vi "configuration UI.vi"() -> ()   [LabVIEW 2013, in "TDMS datalogger editor node.lvclass"]
uses:
  TDMS datalogger editor node.lvclass
  <vilib>/CEF_TreeControl/Node/NodeRef.ctl
  <vilib>/CEF_TreeControl/Node/NISE_CEF_Node.lvclass
  <vilib>/NI/AMC/Message Queue.ctl
  <vilib>/NI/AMC/Message.ctl
  <vilib>/NI/Tools/Keyed Array/KeyedArray.ctl
  <vilib>/CEF_TreeControl/Node/UserEventRef.ctl
  <vilib>/CEF_TreeControl/Controls/EventCluster.ctl
  <vilib>/NI/TBM Modules/TDMS Datalogger/module/configuration/TDMS datalogger configuration.lvclass
  <vilib>/NI/Module Execution Interface/Engine Configuration/engine configuration.lvclass
  <vilib>/NI/Tag Bus Data Framework/Configuration Editor/Classes/Engine Parent/Engine Parent Editor Node.lvclass
  <vilib>/NI/Tag Bus/tag/tag descriptor.lvclass
  <vilib>/NI/Tag Bus/tag/Data Type.ctl
  <vilib>/NI/Tag Bus/tag/tag descriptor.lvclass/tag descriptor.ctl
  <vilib>/NI/Tag Bus Module Framework/root configuration/TBM configuration.lvclass/TBM configuration.ctl
  <vilib>/NI/TBM Modules/TDMS Datalogger/module/configuration/TDMS datalogger configuration.lvclass/TDMS datalogger configuration.ctl
  <vilib>/NI/Tag Bus/tag/write tag name.vi
  <vilib>/NI/Tag Bus/tag/write data type.vi
  <vilib>/NI/TBM Modules/TDMS Datalogger/module/configuration/Write scans per write.vi
  <vilib>/NI/TBM Modules/TDMS Datalogger/module/configuration/Write queue size.vi
  <vilib>/NI/TBM Modules/TDMS Datalogger/module/configuration/Write Path.vi
  <vilib>/NI/TBM Modules/TDMS Datalogger/module/configuration/Write backup directory.vi
  <vilib>/NI/TBM Modules/TDMS Datalogger/module/configuration/Write channel pattern matches.vi
  <vilib>/NI/TBM Modules/TDMS Datalogger/module/configuration/Write add enable channel.vi
  <vilib>/NI/Tag Bus Module Framework/root configuration/Read instance name.vi
  <vilib>/NI/TBM Modules/TDMS Datalogger/module/configuration/Read backup directory.vi
  <vilib>/NI/TBM Modules/TDMS Datalogger/module/configuration/Read Path.vi
  <vilib>/NI/TBM Modules/TDMS Datalogger/module/configuration/Read queue size.vi
  <vilib>/NI/TBM Modules/TDMS Datalogger/module/configuration/Read scans per write.vi
  <vilib>/NI/TBM Modules/TDMS Datalogger/module/configuration/Read add enable channel.vi
  <vilib>/NI/TBM Modules/TDMS Datalogger/module/configuration/Read channel pattern matches.vi
  <vilib>/NI/Tag Bus Data Framework/Configuration Editor/Classes/Module editor node/Read Module Configuration.vi
  <vilib>/NI/Tag Bus Module Framework/root configuration/create GUID.vi
  <vilib>/NI/Tag Bus Data Framework/Configuration Editor/Classes/Module editor node/Write Module Configuration.vi
  <vilib>/NI/Tag Bus Data Framework/Configuration Editor/Classes/Engine Parent/write engine configuration.vi
  <vilib>/NI/Tag Bus Module Framework/root configuration/TBM configuration.lvclass
  <vilib>/NI/Tag Bus Module Framework/module configuration/TBM module configuration.lvclass
  <vilib>/NI/Tag Bus Data Framework/Configuration Editor/Classes/Module editor node/module editor node.lvclass
  <vilib>/CEF_TreeControl/NISE_CEF_TreeControl.lvlib
  <vilib>/NI/Tools/Keyed Array/Tools_KeyedArray.lvlib
  <vilib>/NI/AMC/AMC.lvlib
panel:
  in  "Tab Control":T1(tab)
  in  "channels":i32(listbox)
  in  "remove":bool
  in  "avail tags":i32(listbox)=-1
  in  "add all":bool
  in  "add1":bool
  out "Enable Tag":string
  in  "history error":bool
  in  "path error":bool
  in  "Historical Directory":path
  in  "use enable channel":bool
  in  "recalc":bool
  out "Approximate memory usage":dbl
  in  "queue size":i32=2
  in  "scans per write":i32=20
  in  "File Path":path
  in  "Channel Subscription Pattern Matches":string[](array[string])
  in  "Enable Dynamic Mapping":bool
  in  "user event":T2
  in  "main queue":T3
  in  "node ref":T4
  # "kB"
  # "Note: This value ignores dynamic mapping"
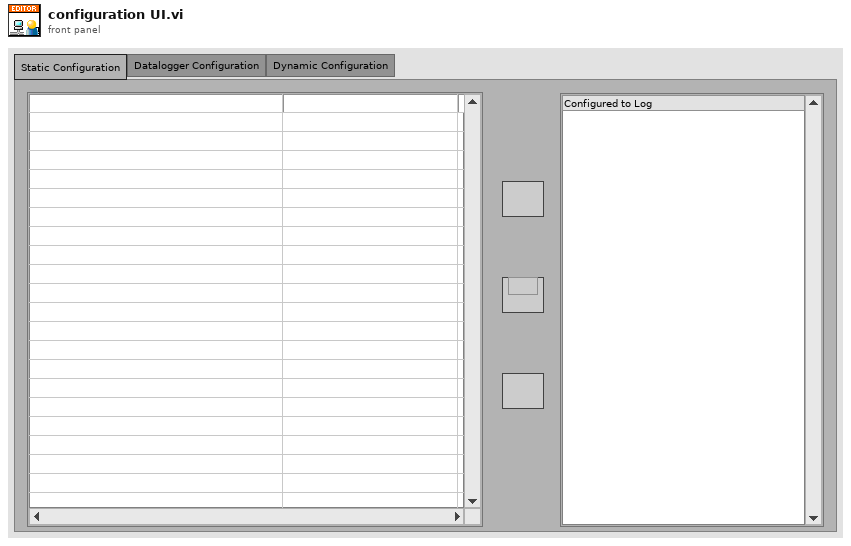
[diagram p1: front panel]
types:
  T1 = enum32{"Static Configuration", "Datalogger Configuration", "Dynamic Configuration"}
  T2 = typedef "NISE_CEF_Node.lvclass/UserEventRef.ctl" = refnum<user-event>
  T3 = typedef "AMC.lvlib/Message Queue.ctl" = refnum<queue>
  T4 = typedef "NISE_CEF_Node.lvclass/NodeRef.ctl" = refnum<data-value>
  T5 = typedef "tag bus.lvlib/tag descriptor.lvclass/Data Type.ctl" = enum16{"Double", "Single", "I64", "I32", "I16", "I8", "U64", "U32", "U16", "U8", "Boolean", "String", "Array of Double", "Array of Single", "Array of I64", "Array of I32", "Array of I16", "Array of I8", "Array of U64", "Array of U32", "Array of U16", "Array of U8", "Array of Boolean", "Array of String"}
  T6 = typedef "NISE_CEF_TreeControl.lvlib/EventCluster.ctl" = cluster{"command":string, "data":string}
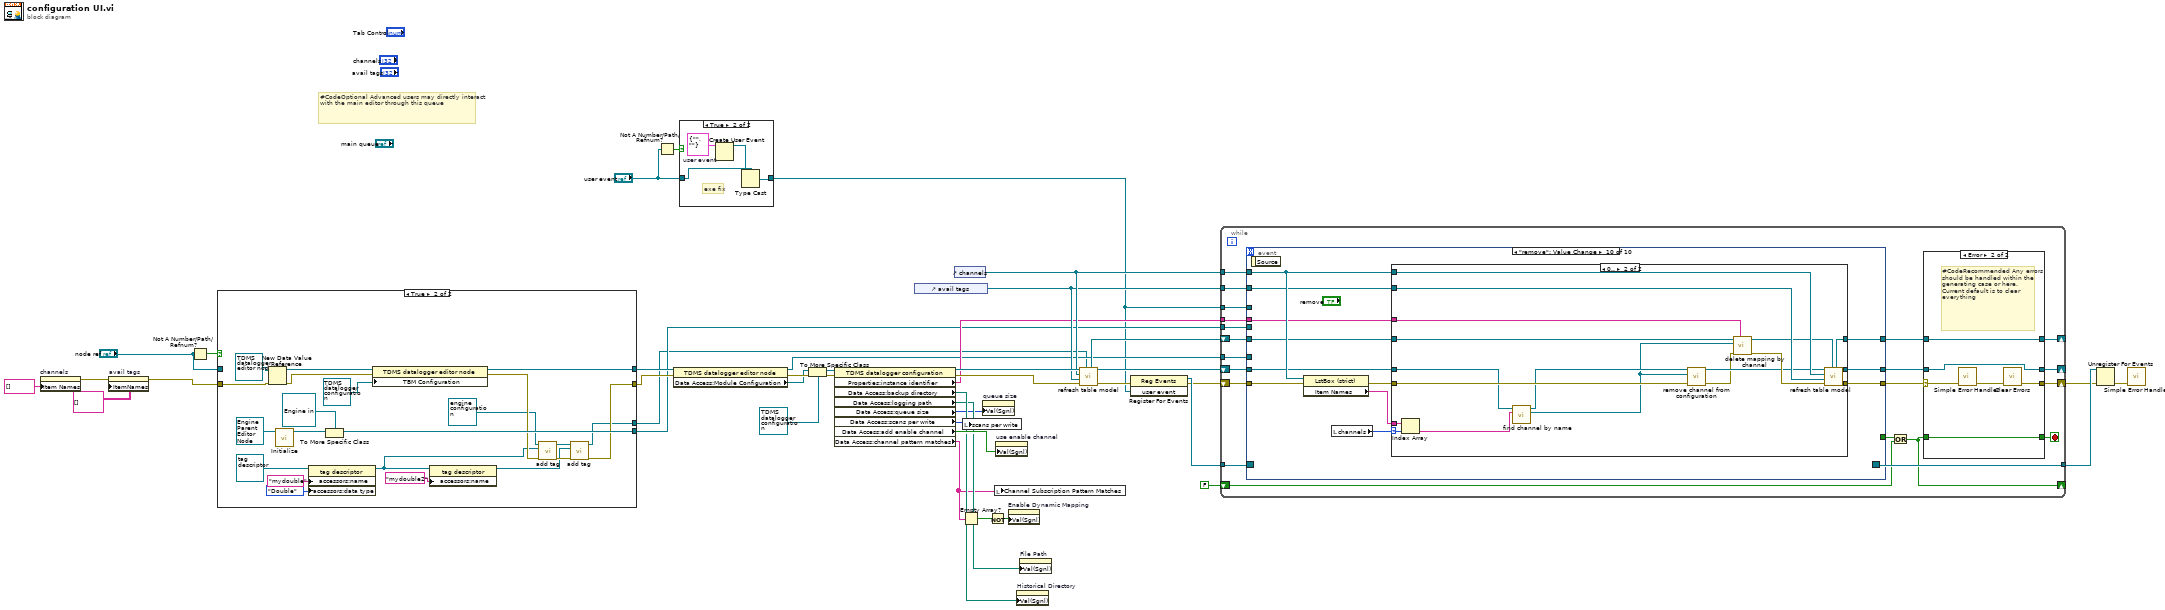
[diagram p0: block diagram]
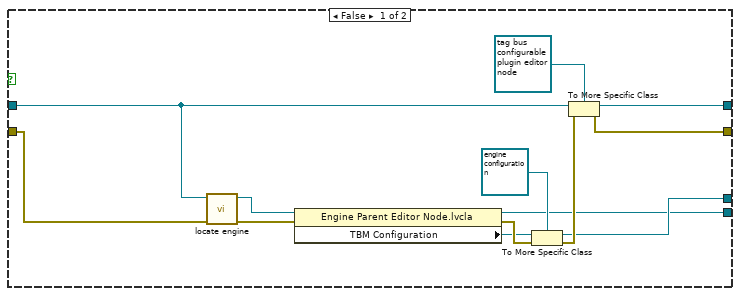
[diagram p2: hidden frame]
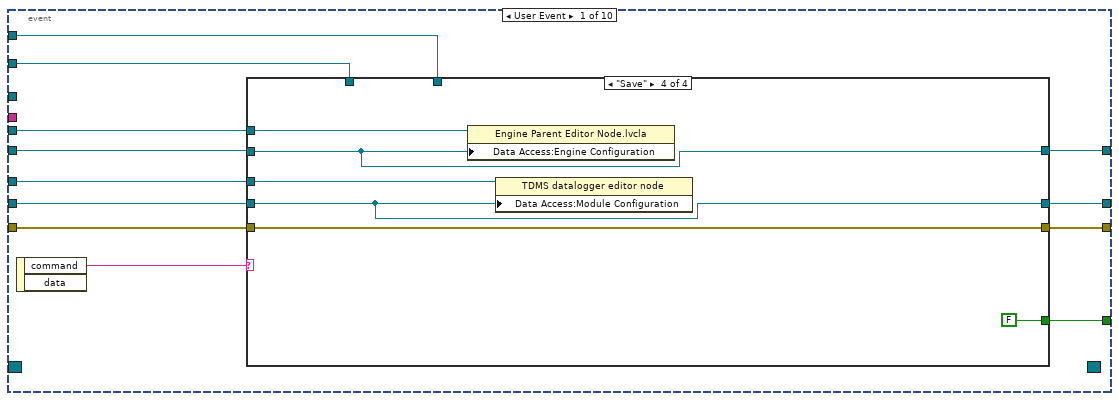
[diagram p5: hidden frame]
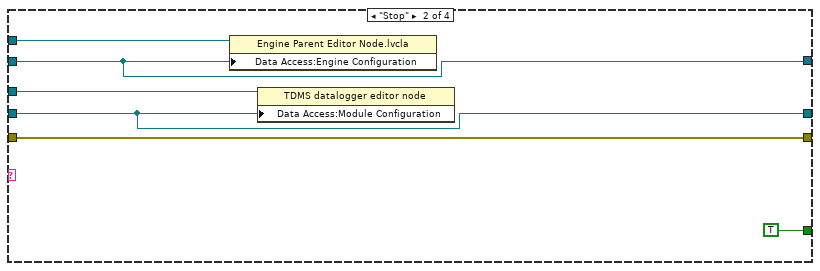
[diagram p7: hidden frame]
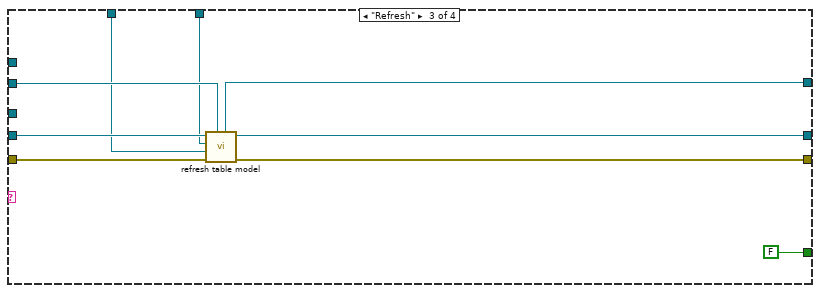
[diagram p8: hidden frame]
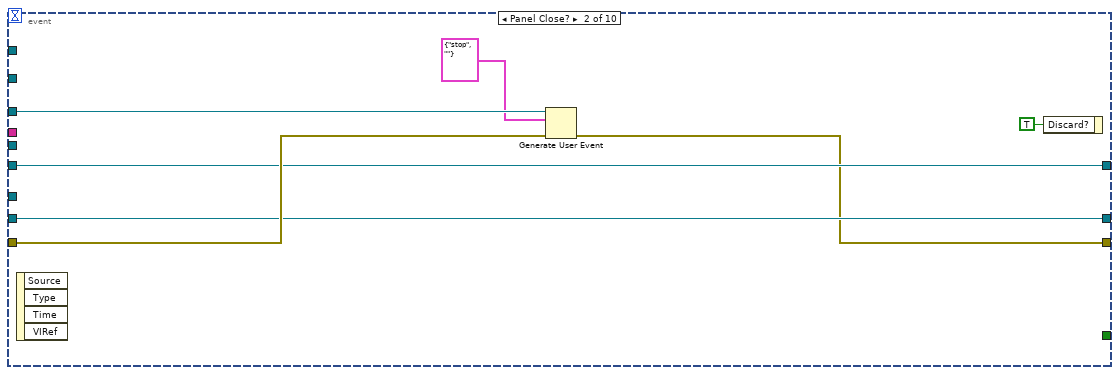
[diagram p9: hidden frame]
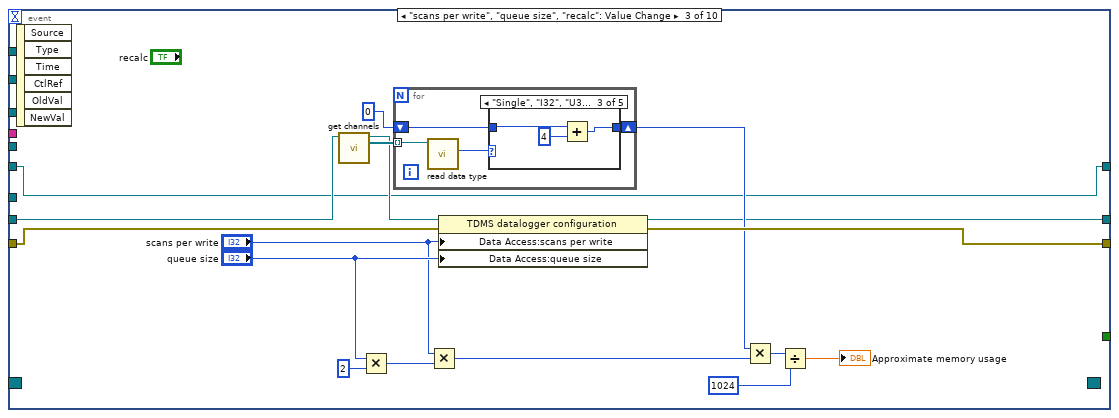
[diagram p10: hidden frame]
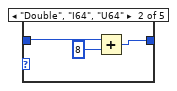
[diagram p12: hidden frame]
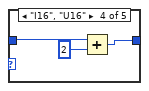
[diagram p13: hidden frame]
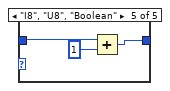
[diagram p14: hidden frame]
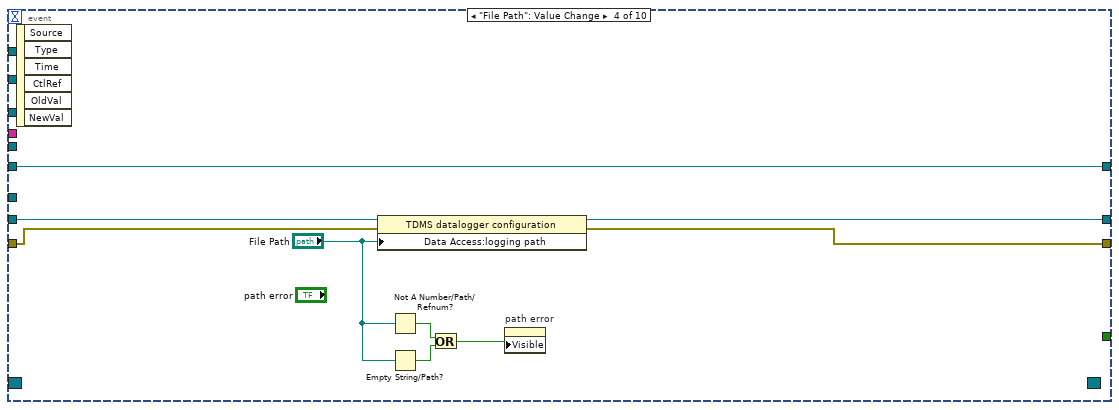
[diagram p15: hidden frame]
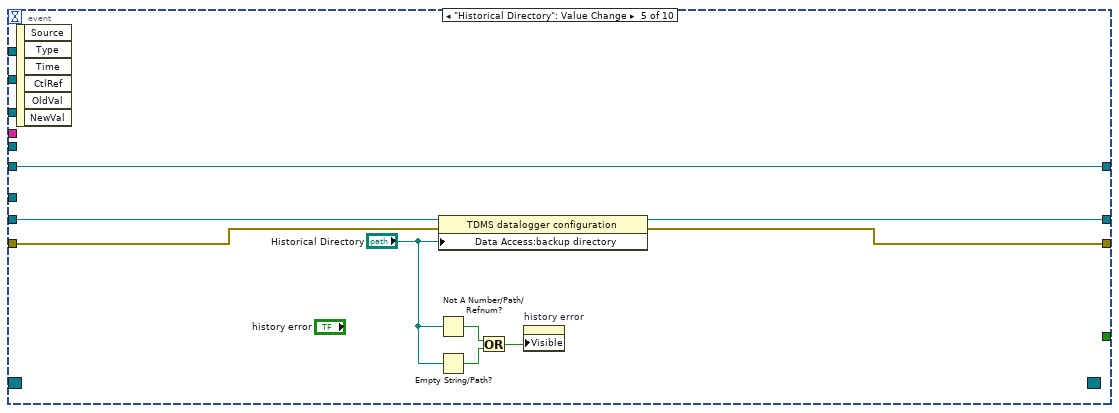
[diagram p16: hidden frame]
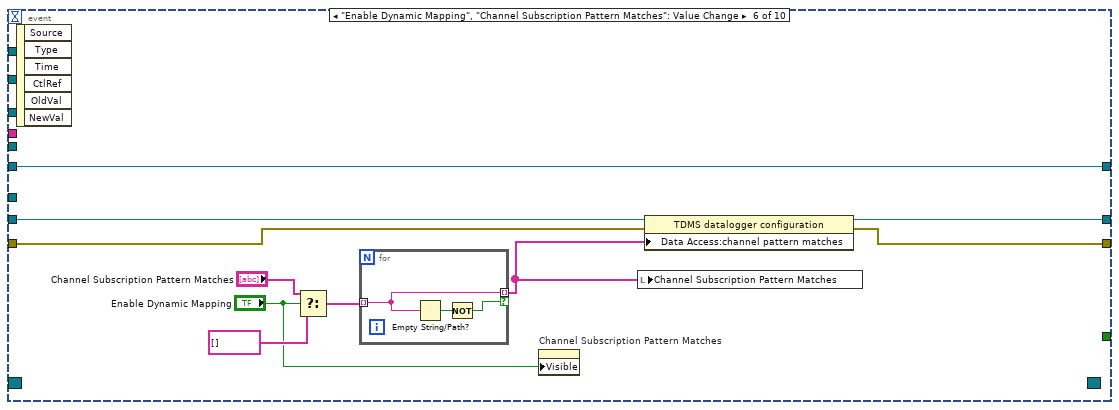
[diagram p17: hidden frame]
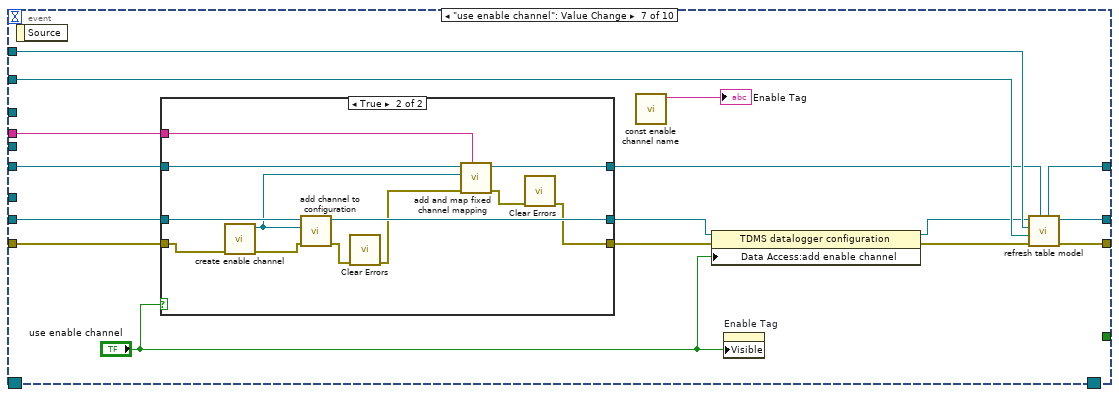
[diagram p18: hidden frame]
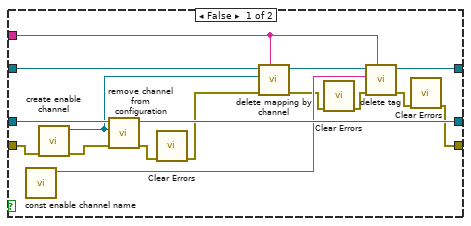
[diagram p19: hidden frame]
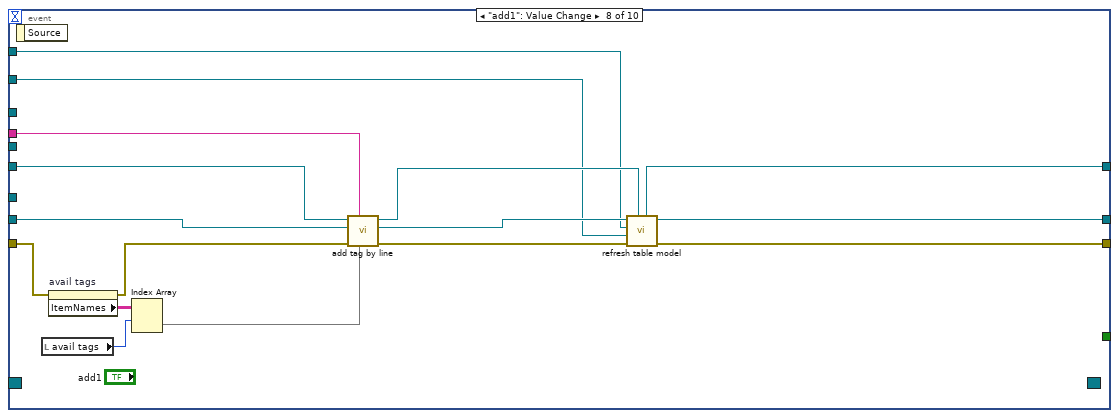
[diagram p20: hidden frame]
diagram:
  # "#CodeOptional Advanced users may directly interact with the main editor through this queue"
  n1 = property on="channels" class="LstBox (strict)"("Item Names"=string[] []) -> (error out=w15:errorcluster)  [unwired: 2 in, 1 out]
  n2 = property on="avail tags" class="MCListbox (strict)"(error in=w15, "ItemNames"=string[][] [] ("Item Names")) -> (error out=w4:errorcluster)  [unwired: 1 in, 1 out]
  n3 = Not A Number/Path/Refnum?(number/path/refnum="node ref") -> (NaN/Path/Refnum?=w6:bool)
  n4 = case shown="True" w6 {
    tunnel: "node ref" -> [w53 _]
    tunnel: [w52 w76] -> w8
    tunnel: [w51 w63] -> w7
    tunnel: [w44 w62] -> w2
    tunnel: [w43 w73] -> w3
    tunnel: w4 -> [w42 w55]
    frame False {
      n5 = call <vilib>:"locate engine.vi"("error in"=w42, "component"=w53) -> ("error out"=w48:errorcluster, "engine"=w50:refnum<data-value>)  [unwired: 8 in]
      n6 = property class="Engine Parent Editor Node.lvcla"(reference=w50, error in=w48) -> (reference out=w43:refnum<data-value>, error out=w47:errorcluster, "TBM Configuration"=w46:refnum<class "TBM configuration.lvclass">)
      n7 = To More Specific Class(target class=refnum<class "engine configuration.lvclass"> refnum ("engine configuration.lvclass"), reference=w46, error in=w47) -> (specific class reference=w44:refnum<class "engine configuration.lvclass">, error out=w45:errorcluster)
      n8 = To More Specific Class(target class=refnum<data-value> refnum ("data value reference"), reference=w53, error in=w45) -> (specific class reference=w52:refnum<data-value>, error out=w51:errorcluster)
    }
    frame True {
      n9 = New Data Value Reference(data value=refnum<class "TDMS datalogger editor node.lvclass"> refnum ("tag bus configurable plugin editor node"), error in=w55) -> (data value reference=w75:refnum<data-value>, error out=w56:errorcluster)
      n10 = call-dynamic "Initialize.vi"("Engine in"=refnum<class "Engine Parent Editor Node.lvclass"> refnum) -> ("data value reference"=w74:T4)  [unwired: 8 in, 2 out]
      n11 = property class="tag descriptor"(reference=refnum<class "tag descriptor.lvclass"> refnum ("tag descriptor"), "accessors:name"="mydouble" ("name"), "accessors:data type"=Data_Type."Double" ("data type")) -> (reference out=w60:refnum<class "tag descriptor.lvclass">)  [unwired: 1 in, 1 out]
      n12 = To More Specific Class(target class=refnum<data-value> refnum ("data value reference"), reference=w74) -> (specific class reference=w73:refnum<data-value>)  [unwired: 1 in, 1 out]
      n13 = property class="TDMS datalogger editor node"(reference=w75, error in=w56, "TBM Configuration"=refnum<class "TDMS datalogger configuration.lvclass"> refnum ("TDMS datalogger configuration")) -> (reference out=w76:refnum<data-value>, error out=w67:errorcluster)
      n14 = property class="tag descriptor"(reference=w60, "accessors:name"="mydouble2" ("name")) -> (reference out=w61:refnum<class "tag descriptor.lvclass">)  [unwired: 1 in, 1 out]
      n15 = call <vilib>:"add tag.vi"("error in"=w67, "tag descriptor"=w60, "engine configuration in"=refnum<class "engine configuration.lvclass"> refnum ("Engine Configuration")) -> ("error out"=w65:errorcluster, "engine configuration out"=w64:refnum<class "engine configuration.lvclass">)  [unwired: 7 in]
      n16 = call <vilib>:"add tag.vi"("error in"=w65, "tag descriptor"=w61, "engine configuration in"=w64) -> ("error out"=w63:errorcluster, "engine configuration out"=w62:refnum<class "engine configuration.lvclass">)  [unwired: 7 in]
    }
  }
  n17 = Not A Number/Path/Refnum?(number/path/refnum="user event") -> (NaN/Path/Refnum?=w10:bool)
  n18 = property class="TDMS datalogger editor node"(reference=w8, error in=w7) -> (reference out=w11:refnum<data-value>, error out=w36:errorcluster, "Data Access:Module Configuration"=w26:refnum<class "TBM module configuration.lvclass">)
  n19 = case shown="True" w10 {
    tunnel: [w77 w80] -> w1
    tunnel: "user event" -> [w77 w81]
    frame False {
    }
    frame True {
      w78 = T6 {"command"="", "data"=""}  # user event
      # "exe fix"
      n20 = Create User Event(user event datatype=w78) -> (user event=w79:refnum<user-event>)  [unwired: 1 in, 1 out]
      n21 = Type Cast(type=w81, x=w79) -> (*(type *) &x=w80:T2)
    }
  }
  n22 = To More Specific Class(target class=refnum<class "TDMS datalogger configuration.lvclass"> refnum ("TDMS datalogger configuration"), reference=w26, error in=w36) -> (specific class reference=w24:refnum<class "TDMS datalogger configuration.lvclass">, error out=w27:errorcluster)
  n23 = property class="TDMS datalogger configuration"(reference=w24, error in=w27) -> (reference out=w20:refnum<class "TDMS datalogger configuration.lvclass">, error out=w19:errorcluster, "Properties:instance identifier"=w16:string, "Data Access:backup directory"=w33:path, "Data Access:logging path"=w32:path, "Data Access:queue size"=w31:i32, "Data Access:scans per write"=w35:i32, "Data Access:add enable channel"=w34:bool, "Data Access:channel pattern matches"=w30:string[])
  n24 = control-ref of="avail tags"() -> (w17:refnum<vi>)
  n25 = control-ref of="channels"() -> (w18:refnum<vi>)
  n26 = Empty Array?(array=w30) -> (empty?=w28:bool)
  n27 = local write "scans per write"(w35) -> ()
  n28 = property on="queue size" class="DigNum (strict)"("Val(Sgnl)"=w31) -> ()  [unwired: 2 in, 2 out]
  n29 = Not(x=w28) -> (.not. x?=w29:bool)
  n30 = local write "Channel Subscription Pattern Matches"(w30) -> ()
  n31 = property on="use enable channel" class="Bool (strict)"("Val(Sgnl)"=w34) -> ()  [unwired: 2 in, 2 out]
  n32 = property on="Enable Dynamic Mapping" class="Bool (strict)"("Val(Sgnl)"=w29) -> ()  [unwired: 2 in, 2 out]
  n33 = property on="Historical Directory" class="Path"("Val(Sgnl)"=w33) -> ()  [unwired: 2 in, 2 out]
  n34 = property on="File Path" class="Path"("Val(Sgnl)"=w32) -> ()  [unwired: 2 in, 2 out]
  n35 = call "refresh table model.vi"("engine configuration"=w2, "error in"=w19, "avail tags"=w17, "chan table"=w18, "TDMS datalogger configuration"=w20) -> ("error out"=w23:errorcluster, "TDMS datalogger configuration out"=w22:refnum<class "TDMS datalogger configuration.lvclass">, "engine configuration out"=w21:refnum<class "engine configuration.lvclass">)  [unwired: 4 in]
  n36 = register-events(error in=w23, w1) -> (reference out=w41:refnum<event-registration>, error out=w38:errorcluster)  [unwired: 1 in]
  n37 = while {
    tunnel: w41 -> [w102]
    tunnel: [w101] -> w40
    shift-right: [w94] -> w12
    shift-left: w38 -> [w100]
    shift-right: [w96] -> _
    shift-left: FALSE -> [w95]
    shift-right: [w91] -> _
    shift-left: w22 -> [w93]
    shift-right: [w89] -> _
    shift-left: w21 -> [w90]
    tunnel: w18 -> [w87]
    tunnel: w17 -> [w86]
    tunnel: w16 -> [w85]
    tunnel: w3 -> [w84]
    tunnel: w11 -> [w83]
    tunnel: w1 -> [w82]
    stop <- w98 stop-if-true
    n38 = event shown="[9] \"remove\": Value Change" {
      selector: w102 -> [_ _ _ _ _ _ _ _ _ _]
      dyn-events: [_ _ _ _ _ _ _ _ _ _] -> w101
      timeout: _ -> [_ _ _ _ _ _ _ _ _ _]
      tunnel: [w124 _ _ _ _ _ _ _ _ _] -> w97
      tunnel: [w122 w151 w171 w196 w205 w215 w236 w275 w290 w314] -> w99
      tunnel: w100 -> [w121 w155 w172 w198 w207 w217 w224 w280 w292 w313]
      tunnel: w93 -> [w119 w154 w159 w197 w206 w216 w225 w265 w291 w304]
      tunnel: [w115 w154 w157 w191 w200 w211 w235 w274 w286 w307] -> w92
      tunnel: [w116 w153 w156 w190 w199 w210 w234 w273 w287 w306] -> w88
      tunnel: w90 -> [w120 w153 w156 w190 w199 w210 w227 w267 w283 w308]
      tunnel: w87 -> [w114 _ _ _ _ _ w233 w270 w284 w311]
      tunnel: w86 -> [w113 _ _ _ _ _ w232 w269 w285 w310]
      tunnel: w85 -> [_ _ _ _ _ _ w229 w268 w281 w305]
      tunnel: w84 -> [w118 _ _ _ _ _ _ _ _ _]
      tunnel: w83 -> [w117 _ _ _ _ _ _ _ _ _]
      tunnel: w82 -> [_ w150 _ _ _ _ _ _ _ _]
      event User Event {
        n39 = event-data() -> ("command"=w123:string)  [unwired: 1 in, 1 out]
        n40 = case shown="\"Save\"" w123 {
          tunnel: [_ TRUE FALSE FALSE] -> w124
          tunnel: [w127 w132 w140 w147] -> w122
          tunnel: w121 -> [w127 w132 w141 w147]
          tunnel: w120 -> [w126 w131 w139 w146]
          tunnel: w119 -> [w125 w130 w137 w145]
          tunnel: w118 -> [_ w128 _ w143]
          tunnel: w117 -> [_ w129 _ w144]
          tunnel: [w126 w131 w138 w146] -> w116
          tunnel: [w125 w130 w136 w145] -> w115
          tunnel: w114 -> [_ _ w135 _]
          tunnel: w113 -> [_ _ w134 _]
          frame Default {
          }
          frame "Stop" {
            n41 = property class="Engine Parent Editor Node.lvcla"(reference=w128, "Data Access:Engine Configuration"=w131) -> ()  [unwired: 1 in, 2 out]
            n42 = property class="TDMS datalogger editor node"(reference=w129, "Data Access:Module Configuration"=w130) -> ()  [unwired: 1 in, 2 out]
          }
          frame "Refresh" {
            n43 = call "refresh table model.vi"("engine configuration"=w139, "error in"=w141, "avail tags"=w134, "chan table"=w135, "TDMS datalogger configuration"=w137) -> ("error out"=w140:errorcluster, "TDMS datalogger configuration out"=w136:refnum<class "TDMS datalogger configuration.lvclass">, "engine configuration out"=w138:refnum<class "engine configuration.lvclass">)  [unwired: 4 in]
          }
          frame "Save" {
            n44 = property class="Engine Parent Editor Node.lvcla"(reference=w143, "Data Access:Engine Configuration"=w146) -> ()  [unwired: 1 in, 2 out]
            n45 = property class="TDMS datalogger editor node"(reference=w144, "Data Access:Module Configuration"=w145) -> ()  [unwired: 1 in, 2 out]
          }
        }
      }
      event Panel Close? {
        n46 = event-data() -> ()  [unwired: 1 in, 4 out]
        n47 = Generate User Event(user event=w150, event data cluster=T6 {"command"="stop", "data"=""} ("event data"), error in=w155) -> (error out=w151:errorcluster)  [unwired: 1 in, 1 out]
        n48 = event-data("Discard?"=TRUE) -> ()  [unwired: 1 in, 1 out]
      }
      event "scans per write", "queue size", "recalc": Value Change {
        n49 = event-data() -> ()  [unwired: 1 in, 6 out]
        n50 = call-dynamic "get channels.vi"("module configuration in"=w159) -> ("channels"=w161:refnum<class "TBM channel.lvclass">[], "module configuration out"=w158:refnum<class "TDMS datalogger configuration.lvclass">)  [unwired: 9 in]
        n51 = Multiply(x="queue size", y=2 ("x")) -> (x*y=w170:i32)
        n52 = for {
          shift-right: [w175] -> w162
          shift-left: u32 0 -> [w176]
          tunnel: w161 -> [w173] mode=indexing
          n53 = call <vilib>:"read data type.vi"("system tag in"=w173) -> ("data type"=w174:T5)  [unwired: 8 in, 2 out]
          n54 = case shown="\"Single\", \"I32\", \"U32\"" w174 {
            tunnel: w176 -> [w177 w180 w183 w186 w189]
            tunnel: [w177 w179 w182 w185 w188] -> w175
            frame Default {
            }
            frame "Double", "I64", "U64" {
              n55 = Add(x=w180, y=u32 8) -> (x+y=w179:u32)
            }
            frame "Single", "I32", "U32" {
              n56 = Add(x=w183, y=u32 4) -> (x+y=w182:u32)
            }
            frame "I16", "U16" {
              n57 = Add(x=w186, y=u32 2) -> (x+y=w185:u32)
            }
            frame "I8", "U8", "Boolean" {
              n58 = Add(x=w189, y=u32 1) -> (x+y=w188:u32)
            }
          }
        }
        n59 = Multiply(x="scans per write", y=w170) -> (x*y=w164:i32)
        n60 = property class="TDMS datalogger configuration"(reference=w158, error in=w172, "Data Access:scans per write"="scans per write", "Data Access:queue size"="queue size") -> (reference out=w157:refnum<class "TDMS datalogger configuration.lvclass">, error out=w171:errorcluster)
        n61 = Multiply(x=w162, y=w164) -> (x*y=w166:u32)
        n62 = Divide(x=w166, y=u32 1024) -> (x/y=→"Approximate memory usage":dbl)
      }
      event "File Path": Value Change {
        n63 = event-data() -> ()  [unwired: 1 in, 6 out]
        n64 = property class="TDMS datalogger configuration"(reference=w197, error in=w198, "Data Access:logging path"="File Path") -> (reference out=w191:refnum<class "TDMS datalogger configuration.lvclass">, error out=w196:errorcluster)
        n65 = Not A Number/Path/Refnum?(number/path/refnum="File Path") -> (NaN/Path/Refnum?=w193:bool)
        n66 = Empty String/Path?(string/path="File Path") -> (empty?=w194:bool)
        n67 = Or(x=w193, y=w194) -> (x .or. y?=w192:bool)
        n68 = property on="path error" class="Bool"("Visible"=w192) -> ()  [unwired: 2 in, 2 out]
      }
      event "Historical Directory": Value Change {
        n69 = event-data() -> ()  [unwired: 1 in, 6 out]
        n70 = Not A Number/Path/Refnum?(number/path/refnum="Historical Directory") -> (NaN/Path/Refnum?=w203:bool)
        n71 = Empty String/Path?(string/path="Historical Directory") -> (empty?=w204:bool)
        n72 = property class="TDMS datalogger configuration"(reference=w206, error in=w207, "Data Access:backup directory"="Historical Directory") -> (reference out=w200:refnum<class "TDMS datalogger configuration.lvclass">, error out=w205:errorcluster)
        n73 = Or(x=w203, y=w204) -> (x .or. y?=w201:bool)
        n74 = property on="history error" class="Bool"("Visible"=w201) -> ()  [unwired: 2 in, 2 out]
      }
      event "Enable Dynamic Mapping", "Channel Subscription Pattern Matches": Value Change {
        n75 = event-data() -> ()  [unwired: 1 in, 6 out]
        n76 = Select(t="Channel Subscription Pattern Matches", s="Enable Dynamic Mapping", f=string[] []) -> (s? t:f=w209:string[])
        n77 = for {
          tunnel: w209 -> [w220] mode=indexing
          tunnel: [w220] -> w208 mode=indexing if=w218
          n78 = Empty String/Path?(string/path=w220) -> (empty?=w219:bool)
          n79 = Not(x=w219) -> (.not. x?=w218:bool)
        }
        n80 = property on="Channel Subscription Pattern Matches" class="Arr (strict)"("Visible"="Enable Dynamic Mapping") -> ()  [unwired: 2 in, 2 out]
        n81 = local write "Channel Subscription Pattern Matches"(w208) -> ()
        n82 = property class="TDMS datalogger configuration"(reference=w216, error in=w217, "Data Access:channel pattern matches"=w208) -> (reference out=w211:refnum<class "TDMS datalogger configuration.lvclass">, error out=w215:errorcluster)
      }
      event "use enable channel": Value Change {
        n83 = event-data() -> ()  [unwired: 1 in, 1 out]
        n84 = case shown="True" "use enable channel" {
          tunnel: w229 -> [w244 w262]
          tunnel: [w245 w263] -> w228
          tunnel: w227 -> [w248 w257]
          tunnel: [w250 w261] -> w226
          tunnel: w225 -> [w251 w260]
          tunnel: w224 -> [w252 w264]
          tunnel: [w239 w255] -> w223
          frame False {
            n85 = call <vilib>:"const enable channel name.vi"() -> ("enable channel"=w243:string)  [unwired: 11 in]
            n86 = call <vilib>:"create enable channel.vi"("error in"=w252) -> ("error out"=w249:errorcluster, "enable channel"=w247:refnum<class "TBM channel.lvclass">)  [unwired: 9 in]
            n87 = call <vilib>:"remove channel from configuration.vi"("error in"=w249, "TBM channel in"=w247, "TDMS datalogger configuration in"=w251) -> ("error out"=w238:errorcluster, "TDMS datalogger configuration out"=w250:refnum<class "TDMS datalogger configuration.lvclass">)  [unwired: 7 in]
            n88 = call <vilib>:"Clear Errors.vi"("error in (no error)"=w238) -> ("error out"=w237:errorcluster)  [unwired: 6 in]
            n89 = call <vilib>:"delete mapping by channel.vi"("owner ID"=w244, "error in"=w237, "channel"=w247, "engine configuration in"=w248) -> ("error out"=w241:errorcluster, "engine configuration out"=w246:refnum<class "engine configuration.lvclass">)  [unwired: 6 in]
            n90 = call <vilib>:"Clear Errors.vi"("error in (no error)"=w241) -> ("error out"=w242:errorcluster)  [unwired: 6 in]
            n91 = call <vilib>:"delete tag.vi"("owner ID"=w244, "error in"=w242, "tag name"=w243, "engine configuration in"=w246) -> ("error out"=w240:errorcluster, "engine configuration out"=w245:refnum<class "engine configuration.lvclass">)  [unwired: 6 in]
            n92 = call <vilib>:"Clear Errors.vi"("error in (no error)"=w240) -> ("error out"=w239:errorcluster)  [unwired: 6 in]
          }
          frame True {
            n93 = call <vilib>:"create enable channel.vi"("error in"=w264) -> ("error out"=w259:errorcluster, "enable channel"=w258:refnum<class "TBM channel.lvclass">)  [unwired: 9 in]
            n94 = call <vilib>:"add channel to configuration.vi"("error in"=w259, "TBM channel in"=w258, "TDMS datalogger configuration in"=w260) -> ("error out"=w254:errorcluster, "TDMS datalogger configuration out"=w261:refnum<class "TDMS datalogger configuration.lvclass">)  [unwired: 7 in]
            n95 = call <vilib>:"Clear Errors.vi"("error in (no error)"=w254) -> ("error out"=w253:errorcluster)  [unwired: 6 in]
            n96 = call <vilib>:"add and map fixed channel mapping.vi"("module instance"=w262, "error in"=w253, "fixed channel"=w258, "engine configuration in"=w257) -> ("error out"=w256:errorcluster, "engine configuration out"=w263:refnum<class "engine configuration.lvclass">)  [unwired: 6 in]
            n97 = call <vilib>:"Clear Errors.vi"("error in (no error)"=w256) -> ("error out"=w255:errorcluster)  [unwired: 6 in]
          }
        }
        n98 = call <vilib>:"const enable channel name.vi"() -> ("enable channel"=→"Enable Tag":string)  [unwired: 11 in]
        n99 = property class="TDMS datalogger configuration"(reference=w226, error in=w223, "Data Access:add enable channel"="use enable channel") -> (reference out=w230:refnum<class "TDMS datalogger configuration.lvclass">, error out=w231:errorcluster)
        n100 = property on="Enable Tag" class="Str"("Visible"="use enable channel") -> ()  [unwired: 2 in, 2 out]
        n101 = call "refresh table model.vi"("engine configuration"=w228, "error in"=w231, "avail tags"=w232, "chan table"=w233, "TDMS datalogger configuration"=w230) -> ("error out"=w236:errorcluster, "TDMS datalogger configuration out"=w235:refnum<class "TDMS datalogger configuration.lvclass">, "engine configuration out"=w234:refnum<class "engine configuration.lvclass">)  [unwired: 4 in]
      }
      event "add1": Value Change {
        n102 = event-data() -> ()  [unwired: 1 in, 1 out]
        n103 = local read "avail tags"() -> (w278:i32)
        n104 = property on="avail tags" class="MCListbox (strict)"(error in=w280) -> (error out=w277:errorcluster, "ItemNames"=w279:string[][])  [unwired: 1 in, 1 out]
        n105 = Index Array(array=w279, index (row)=w278) -> (element=w266:string[])  [unwired: 1 in]
        n106 = call "add tag by line.vi"("ItemNames"=w266, "Properties:instance identifier"=w268, "error in"=w277, "TDMS datalogger configuration in"=w265, "engine configuration in"=w267) -> ("error out"=w276:errorcluster, "TDMS datalogger configuration out"=w271:refnum<class "TDMS datalogger configuration.lvclass">, "engine configuration out"=w272:refnum<class "engine configuration.lvclass">)  [unwired: 4 in]
        n107 = call "refresh table model.vi"("engine configuration"=w272, "error in"=w276, "avail tags"=w269, "chan table"=w270, "TDMS datalogger configuration"=w271) -> ("error out"=w275:errorcluster, "TDMS datalogger configuration out"=w274:refnum<class "TDMS datalogger configuration.lvclass">, "engine configuration out"=w273:refnum<class "engine configuration.lvclass">)  [unwired: 4 in]
      }
      event "add all": Value Change {
        n108 = event-data() -> ()  [unwired: 1 in, 1 out]
        n109 = property on="avail tags" class="MCListbox (strict)"(error in=w292) -> (error out=w294:errorcluster, "ItemNames"=w293:string[][])  [unwired: 1 in, 1 out]
        n110 = for {
          tunnel: w293 -> [w295] mode=indexing
          shift-right: [w301] -> w289
          shift-left: w294 -> [w299]
          shift-right: [w302] -> w288
          shift-left: w291 -> [w300]
          shift-right: [w297] -> w282
          shift-left: w283 -> [w298]
          tunnel: w281 -> [w296]
          n111 = call "add tag by line.vi"("ItemNames"=w295, "Properties:instance identifier"=w296, "error in"=w299, "TDMS datalogger configuration in"=w300, "engine configuration in"=w298) -> ("error out"=w301:errorcluster, "TDMS datalogger configuration out"=w302:refnum<class "TDMS datalogger configuration.lvclass">, "engine configuration out"=w297:refnum<class "engine configuration.lvclass">)  [unwired: 4 in]
        }
        n112 = call "refresh table model.vi"("engine configuration"=w282, "error in"=w289, "avail tags"=w285, "chan table"=w284, "TDMS datalogger configuration"=w288) -> ("error out"=w290:errorcluster, "TDMS datalogger configuration out"=w286:refnum<class "TDMS datalogger configuration.lvclass">, "engine configuration out"=w287:refnum<class "engine configuration.lvclass">)  [unwired: 4 in]
      }
      event "remove": Value Change {
        n113 = event-data() -> ()  [unwired: 1 in, 1 out]
        n114 = property class="LstBox (strict)"(reference=w311, error in=w313) -> (error out=w309:errorcluster, "Item Names"=w312:string[])  [unwired: 1 out]
        n115 = local read "channels"() -> (w303:i32)
        n116 = case shown="0.." w303 {
          selector: w303 -> [_ w318]
          tunnel: [w315 w335] -> w314
          tunnel: w312 -> [_ w334]
          tunnel: w311 -> [_ w333]
          tunnel: w310 -> [_ w332]
          tunnel: w309 -> [w315 w331]
          tunnel: w308 -> [w317 w330]
          tunnel: [w316 w327] -> w307
          tunnel: [w317 w325] -> w306
          tunnel: w305 -> [_ w324]
          tunnel: w304 -> [w316 w322]
          frame ..-1 {
          }
          frame 0.. {
            n117 = Index Array(array=w334, index=w318) -> (element=w320:string)
            n118 = call <vilib>:"find channel by name.vi"("channel name"=w320, "TDMS datalogger configuration in"=w322) -> ("channel"=w319:refnum<class "TBM channel.lvclass">, "TDMS datalogger configuration out"=w321:refnum<class "TDMS datalogger configuration.lvclass">)  [unwired: 8 in]
            n119 = call <vilib>:"remove channel from configuration.vi"("error in"=w331, "TBM channel in"=w319, "TDMS datalogger configuration in"=w321) -> ("error out"=w323:errorcluster, "TDMS datalogger configuration out"=w328:refnum<class "TDMS datalogger configuration.lvclass">)  [unwired: 7 in]
            n120 = call <vilib>:"delete mapping by channel.vi"("owner ID"=w324, "error in"=w323, "channel"=w319, "engine configuration in"=w330) -> ("error out"=w329:errorcluster, "engine configuration out"=w326:refnum<class "engine configuration.lvclass">)  [unwired: 6 in]
            n121 = call "refresh table model.vi"("engine configuration"=w326, "error in"=w329, "avail tags"=w332, "chan table"=w333, "TDMS datalogger configuration"=w328) -> ("error out"=w335:errorcluster, "TDMS datalogger configuration out"=w327:refnum<class "TDMS datalogger configuration.lvclass">, "engine configuration out"=w325:refnum<class "engine configuration.lvclass">)  [unwired: 4 in]
          }
        }
      }
    }
    n122 = Or(x=w97, y=w95) -> (x .or. y?=w96:bool)
    n123 = case shown="Error" w99 {
      selector: w99 -> [w105 w111]
      tunnel: [w106 w112] -> w98
      tunnel: w96 -> [w106 w112]
      tunnel: [w105 w109] -> w94
      tunnel: w92 -> [w104 w108]
      tunnel: [w104 w108] -> w91
      tunnel: [w103 w107] -> w89
      tunnel: w88 -> [w103 w107]
      frame No Error {
      }
      frame Error {
        # "#CodeRecommended Any errors should be handled within the generating case or here. Current default is to clear everything"
        n124 = call <vilib>:"Simple Error Handler.vi"("error in (no error)"=w111) -> ("error out"=w110:errorcluster)  [unwired: 4 in, 4 out]
        n125 = call <vilib>:"Clear Errors.vi"("error in (no error)"=w110) -> ("error out"=w109:errorcluster)  [unwired: 6 in]
      }
    }
  }
  n126 = Unregister For Events(event registration refnum=w40, error in=w12) -> (error out=w37:errorcluster)
  n127 = call <vilib>:"Simple Error Handler.vi"("error in (no error)"=w37) -> ()  [unwired: 4 in, 5 out]
